vi "Adj Data buffer.vi"(7 "buffer size":i32=30, 11 "data buffer":i32[](array[numeric])) -> (3 "data buffer out":i32[](array[numeric]))   [LabVIEW 2018]
doc: "将数据源按照预定的大小进行取样调整（默认取样空间大小30）"
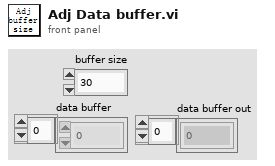
[diagram p1: front panel]
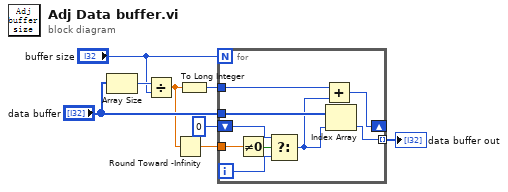
[diagram p0: block diagram]
diagram:
  n1 = Array Size(array="data buffer") -> (size(s)=w8:i32)
  n2 = Divide(x=w8, y="buffer size") -> (x/y=w2:dbl)
  n3 = Round Toward -Infinity(1:w2) -> (0:w1:dbl)
  n4 = To Long Integer(number=w2) -> (32bit integer=w6:i32)
  n5 = for {
    N: "buffer size" -> [_]
    tunnel: "data buffer" -> [w17]
    tunnel: w6 -> [w9]
    shift-right: [w16] -> _
    shift-left: 0 -> [w12]
    tunnel: [w15] -> w4 mode=indexing
    tunnel: w1 -> [w14]
    i -> [w11]
    n6 = Not Equal To 0?(x=w14) -> (x != 0?=w13:bool)
    n7 = Select(t=w12, s=w13, f=w11) -> (s? t:f=w10:i32)
    n8 = Add(x=w9, y=w10) -> (x+y=w16:i32)
    n9 = Index Array(array=w17, index=w10) -> (element=w15:i32)
  }
  "data buffer out" <- w4
